vi "Config Write Robot Globals.vi"(11 "refnum":T1) -> (3 "refnum 2":T1)   [LabVIEW 2012]
uses:
  <vilib>/Utility/config.llb/Config Data RefNum.ctl
  Robot Global Data.vi
  <vilib>/Utility/config.llb/Write Key (Double).vi
  <vilib>/Utility/config.llb/NI_LVConfig.lvlib
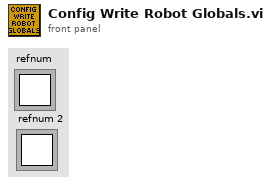
[diagram p1: front panel]
types:
  T1 = typedef "NI_LVConfig.lvlib/Config Data RefNum.ctl" = refnum<k1>
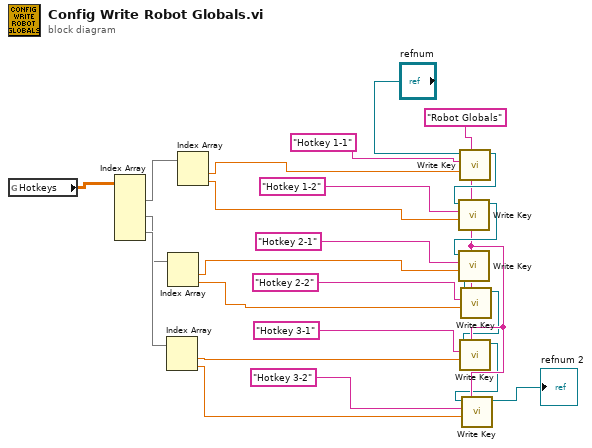
[diagram p0: block diagram]
diagram:
  w6 = "Robot Globals"
  n1 = global read "Robot Global Data.vi" "Hotkeys"() -> (w16:dbl[][])
  n2 = Index Array(array=w16) -> (element #1=w13:dbl[], element #2=w14:dbl[], element #3=w15:dbl[])  [unwired: 6 in]
  n3 = Index Array(array=w15) -> (element #1=w8:dbl, element #2=w7:dbl)  [unwired: 2 in]
  n4 = Index Array(array=w14) -> (element #1=w10:dbl, element #2=w9:dbl)  [unwired: 2 in]
  n5 = Index Array(array=w13) -> (element #1=w12:dbl, element #2=w11:dbl)  [unwired: 2 in]
  n6 = call-poly <vilib>:"Write Key.vi"("section"=w6, "value"=w12, "key"="Hotkey 1-1", "refnum"="refnum") -> ("refnum out"=w23:T1)  [unwired: 5 in, 2 out]
  n7 = call-poly <vilib>:"Write Key.vi"("section"=w6, "value"=w11, "key"="Hotkey 1-2", "refnum"=w23) -> ("refnum out"=w22:T1)  [unwired: 5 in, 2 out]
  n8 = call-poly <vilib>:"Write Key.vi"("section"=w6, "value"=w10, "key"="Hotkey 2-1", "refnum"=w22) -> ("refnum out"=w21:T1)  [unwired: 5 in, 2 out]
  n9 = call-poly <vilib>:"Write Key.vi"("section"=w6, "value"=w9, "key"="Hotkey 2-2", "refnum"=w21) -> ("refnum out"=w3:T1)  [unwired: 5 in, 2 out]
  n10 = call-poly <vilib>:"Write Key.vi"("section"=w6, "value"=w8, "key"="Hotkey 3-1", "refnum"=w3) -> ("refnum out"=w2:T1)  [unwired: 5 in, 2 out]
  n11 = call-poly <vilib>:"Write Key.vi"("section"=w6, "value"=w7, "key"="Hotkey 3-2", "refnum"=w2) -> ("refnum out"=→"refnum 2":T1)  [unwired: 5 in, 2 out]
